vi "INI Tester.vi"() -> ()   [LabVIEW 2013]
uses:
  FA_INIconfig.ctl
  FA_INI.ctl
  FA_LocalStore API/source/VI Source/FA_LSSpecialTypes.ctl
  FA_INI.lvlib
  FA_LocalStore API/source/VI Source/FA_LocalStore.lvlib
panel:
  out "Error Out":errorcluster
  in  "Error In":errorcluster
  out "XML String Output":string
  out "Config":T1
  in  "XML String":string="<?xml version=\"1.0\" encoding=\"UTF-8\"?>\n<Config>\n  <Id>0dac3609-a663-42f1-bc0b-7e1790b8cb89</Id>\n  <Name>New Config</Name>\n  <Type>INI</Type>\n  <INI>\n\t<Destination>ni-rt.ini</Destination>\n\t<Section>\n\t\t<Section_Name>LVRT</Section_Name>\n\t\t<Token>\n\t\t\t<Key>RTTarget.ApplicationPath</Key>\n\t\t\t<Value>/ni-rt/startup/startup.rtexe</Value>\n\t\t</Token>\n\t\t<Token>\n\t\t\t<Key>RTTarget.LaunchAppAtBoot</Key>\n\t\t\t<Value>True</Value>\n\t\t</Token>\n\t</Section>\n  </INI>\n  <INI>\n\t<Destination>ni-rt.ini</Destination>\n\t<Section>\n\t\t<Section_Name>LVRT</Section_Name>\n\t\t<Token>\n\t\t\t<Key>myToken1</Key>\n\t\t\t<Value>True</Value>\n\t\t</Token>\n\t\t<Token>\n\t\t\t<Key>myToken2</Key>\n\t\t\t<Value>False</Value>\n\t\t</Token>\n\t</Section>\n  </INI>\n  <Account>5678</Account>\n  <CreateDate>2012-05-15T19:45:29.275Z</CreateDate>\n  <LastModified>2012-05-15T19:45:29.275Z</LastModified>\n</Config>"
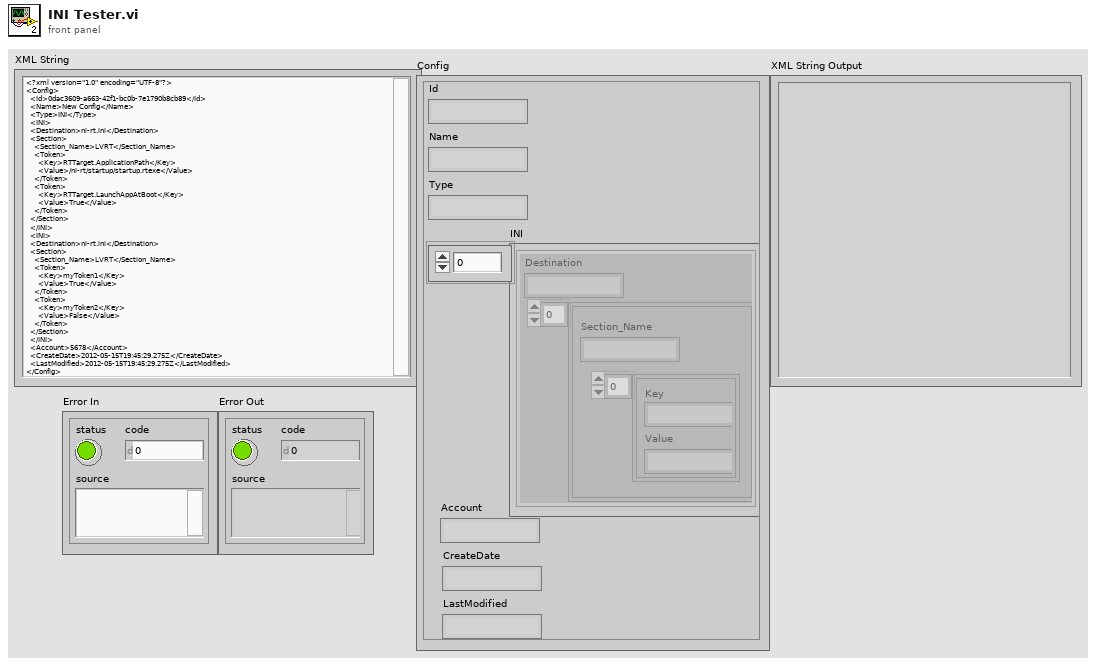
[diagram p1: front panel]
types:
  T1 = typedef "FA_INI.lvlib/FA_INIconfig.ctl" = cluster{"Id":string, "Name":string, "Type":string, "INI":T2, "Account":string, "CreateDate":string, "LastModified":string}
  T2 = typedef "FA_INI.ctl" = cluster{"Destination":string, "Section":cluster{"Section_Name":string, "Token":cluster{"Key":string, "Value":string}[]}[]}[]
  T3 = typedef "FA_LocalStore.lvlib/FA_LSSpecialTypes.ctl" = string
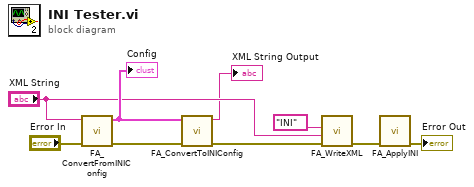
[diagram p0: block diagram]
diagram:
  n1 = call "FA_ConvertFromINIConfig.vi"("Error In"="Error In", "XML String"="XML String") -> ("Error Out"=w7:errorcluster, "Config"=w9:T1)  [unwired: 8 in]
  "Config" <- w9
  n2 = call "FA_ConvertToINIConfig.vi"("Error In"=w7, "Config"=w9) -> ("Error Out"=w6:errorcluster, "XML String"=→"XML String Output":string)  [unwired: 8 in]
  n3 = call "FA_WriteXML.vi"("Error In"=w6, "XML String"="XML String", "Special Type"=T3 "INI") -> ("Error Out"=w3:errorcluster)  [unwired: 6 in]
  n4 = call "FA_ApplyINI.vi"("Error In"=w3) -> ("Error Out"=→"Error Out":errorcluster)  [unwired: 10 in]
